vi "手指弯曲.vi"(8 "error in (no error)":errorcluster caption="错误输入（无错误）", 10 "Hands Data In":T1={"手腕"=254.32835, "小手指"=0.0, "无名指"=0.0, "中指"=0.0, "食指"=61.343285, "上下移动"=-1.8918918918918917, "背景色"=15204350, "拇指"=0.0, "转台"=223.8806, "手臂"=20.597015} {"手臂" scale=0.0..90.0; "转台" scale=0.0..360.0; "拇指" scale=0.0..90.0; "上下移动" scale=0.0..100.0; "食指" scale=0.0..90.0; "中指" scale=0.0..90.0; "无名指" scale=0.0..90.0; "小手指" scale=0.0..90.0; "手腕" scale=0.0..360.0}, 11 "Hands Ref In":T2) -> (0 "error out":errorcluster caption="错误输出", 2 "Hands Data Out":T1={"手腕"=52.38806, "小手指"=0.0, "无名指"=0.0, "中指"=0.0, "食指"=0.0, "上下移动"=-1.8918918918918917, "背景色"=15204350, "拇指"=0.0, "转台"=52.38806, "手臂"=52.38806} {"手臂" scale=0.0..90.0; "转台" scale=0.0..360.0; "拇指" scale=0.0..90.0; "上下移动" scale=0.0..100.0; "食指" scale=0.0..90.0; "中指" scale=0.0..90.0; "无名指" scale=0.0..90.0; "小手指" scale=0.0..90.0; "手腕" scale=0.0..360.0}, 3 "Hands Ref Out":T2)   [LabVIEW 2016]
uses:
  Controls/handdata.ctl
  Controls/robotdata.ctl
  <vilib>/picture/3D Picture Control/NI_3D Picture Control.lvlib
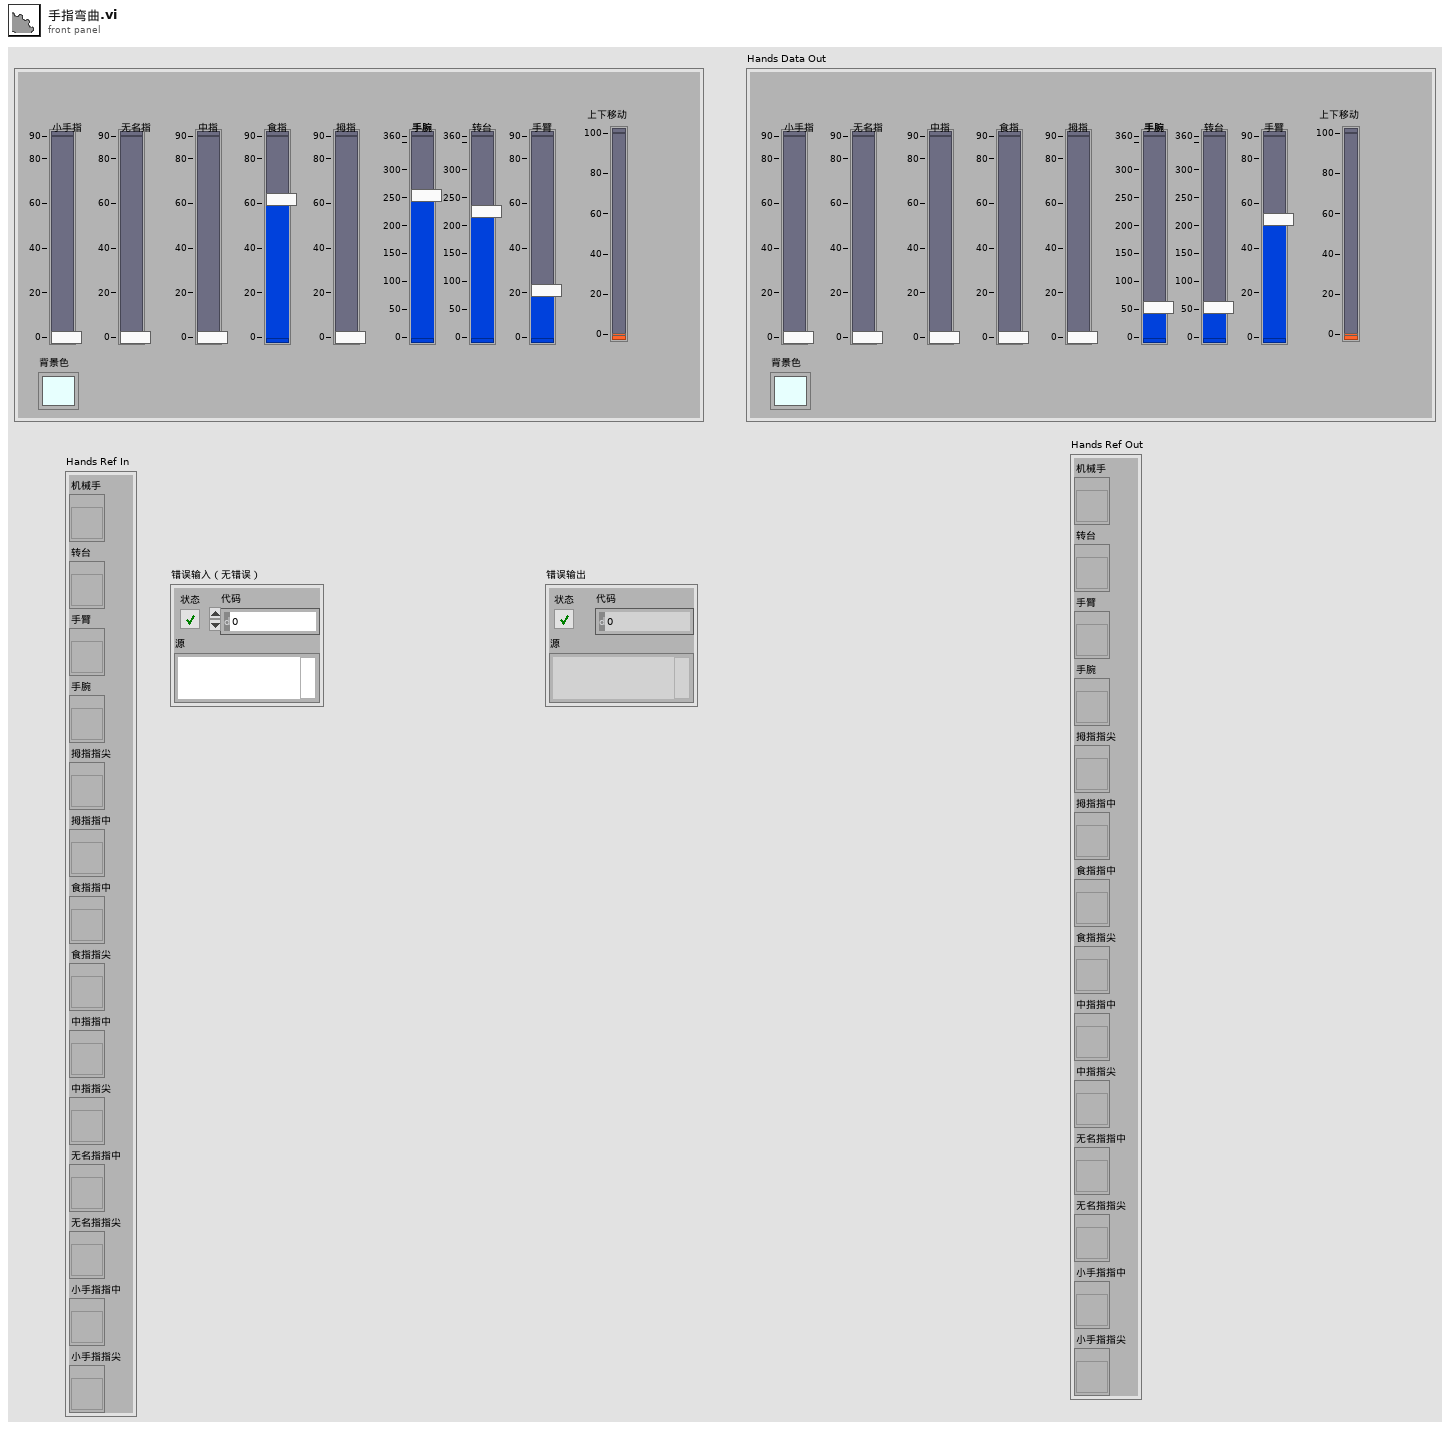
[diagram p1: front panel]
types:
  T1 = typedef "robotdata.ctl" = cluster{"手腕":sgl, "小手指":sgl, "无名指":sgl, "中指":sgl, "食指":sgl, "上下移动":dbl, "背景色":u32, "拇指":sgl, "转台":sgl, "手臂":sgl}
  T2 = typedef "handdata.ctl" = cluster{"机械手":refnum<vi>, "转台":refnum<vi>, "手臂":refnum<vi>, "手腕":refnum<vi>, "拇指指尖":refnum<vi>, "拇指指中 ":refnum<vi>, "食指指中":refnum<vi>, "食指指尖":refnum<vi>, "中指指中":refnum<vi>, "中指指尖":refnum<vi>, "无名指指中":refnum<vi>, "无名指指尖":refnum<vi>, "小手指指中":refnum<vi>, "小手指指尖":refnum<vi>}
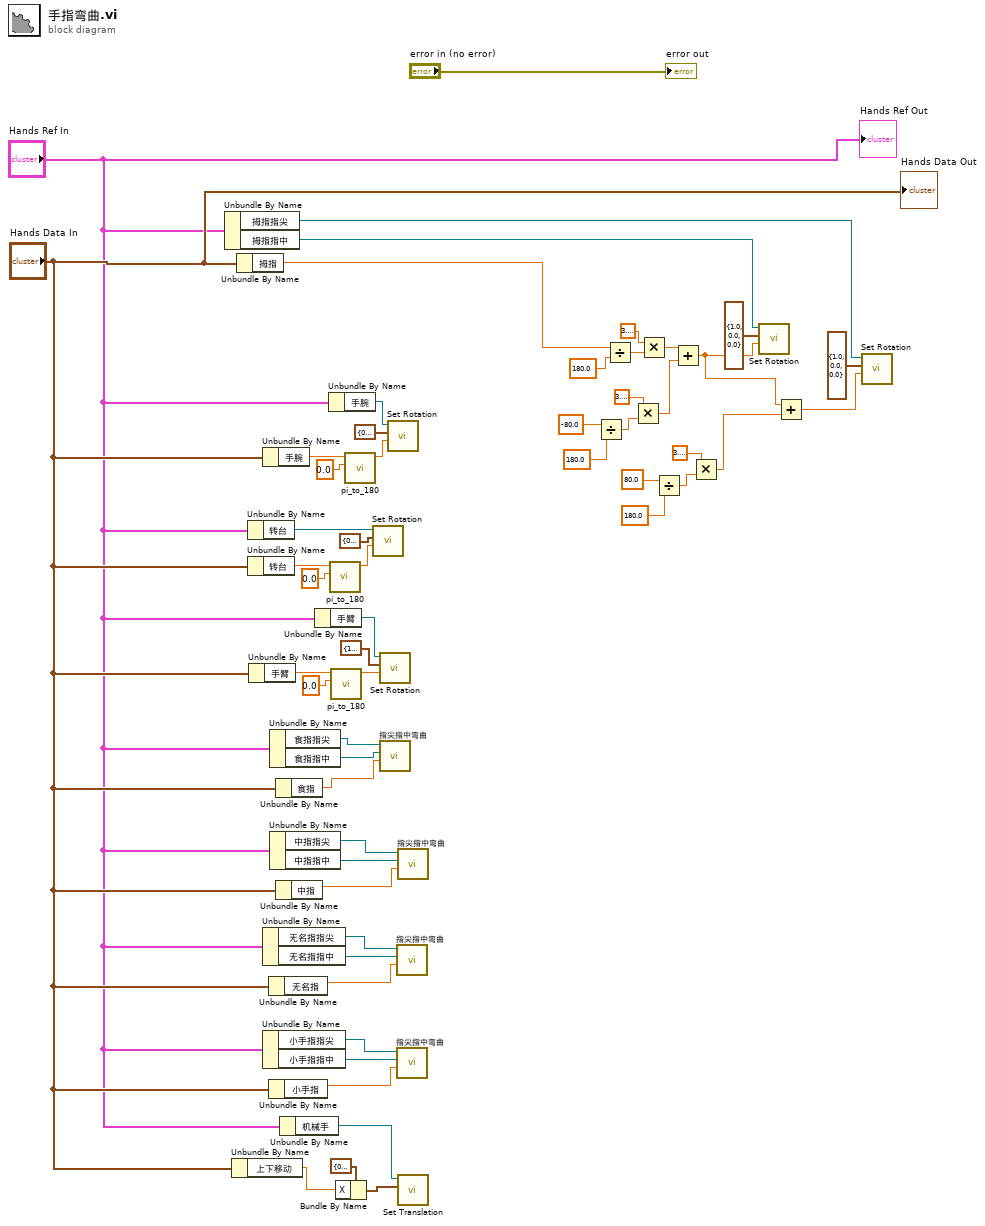
[diagram p0: block diagram]
diagram:
  n1 = Unbundle By Name("Hands Ref In") -> ("拇指指尖"=w10:refnum<vi>, "拇指指中"=w11:refnum<vi>)
  n2 = Unbundle By Name("Hands Data In") -> ("上下移动"=w26:dbl)
  n3 = Unbundle By Name("Hands Data In") -> ("拇指"=w9:sgl)
  n4 = Unbundle By Name("Hands Ref In") -> ("转台"=w49:refnum<vi>)
  n5 = Unbundle By Name("Hands Data In") -> ("转台"=w45:sgl)
  n6 = Unbundle By Name("Hands Data In") -> ("手臂"=w43:sgl)
  n7 = Unbundle By Name("Hands Data In") -> ("手腕"=w51:sgl)
  n8 = Unbundle By Name("Hands Ref In") -> ("无名指指尖"=w34:refnum<vi>, "无名指指中"=w33:refnum<vi>)
  n9 = Unbundle By Name("Hands Ref In") -> ("小手指指尖"=w29:refnum<vi>, "小手指指中"=w30:refnum<vi>)
  n10 = Unbundle By Name("Hands Data In") -> ("无名指"=w32:sgl)
  n11 = Unbundle By Name("Hands Data In") -> ("小手指"=w31:sgl)
  n12 = Unbundle By Name("Hands Ref In") -> ("食指指尖"=w40:refnum<vi>, "食指指中"=w39:refnum<vi>)
  n13 = Unbundle By Name("Hands Ref In") -> ("中指指尖"=w35:refnum<vi>, "中指指中"=w36:refnum<vi>)
  n14 = Unbundle By Name("Hands Data In") -> ("食指"=w38:sgl)
  n15 = Unbundle By Name("Hands Data In") -> ("中指"=w37:sgl)
  n16 = Unbundle By Name("Hands Ref In") -> ("机械手"=w25:refnum<vi>)
  n17 = Unbundle By Name("Hands Ref In") -> ("手臂"=w47:refnum<vi>)
  n18 = Unbundle By Name("Hands Ref In") -> ("手腕"=w52:refnum<vi>)
  n19 = call "pi_to_180.vi"("起始角度"=0.0, "输入角度"=w45) -> ("数值"=w46:dbl)  [unwired: 9 in]
  n20 = call "pi_to_180.vi"("起始角度"=0.0, "输入角度"=w43) -> ("数值"=w41:dbl)  [unwired: 9 in]
  n21 = Bundle By Name(cluster=cluster{"X":sgl, "Y":sgl, "Z":sgl} {"X"=0.0, "Y"=0.0, "Z"=0.0} ("Translation"), "X"=w26) -> (w28:cluster{"X":sgl, "Y":sgl, "Z":sgl})
  n22 = call "pi_to_180.vi"("起始角度"=0.0, "输入角度"=w51) -> ("数值"=w53:dbl)  [unwired: 9 in]
  n23 = call <vilib>:"Set Rotation.vi"("Angle"=w46, "Axis"=cluster{"X":sgl, "Y":sgl, "Z":sgl} {"X"=0.0, "Y"=0.0, "Z"=1.0}, "Scene Object"=w49) -> ()  [unwired: 7 in, 2 out]
  n24 = call <vilib>:"Set Rotation.vi"("Angle"=w41, "Axis"=cluster{"X":sgl, "Y":sgl, "Z":sgl} {"X"=1.0, "Y"=0.0, "Z"=0.0}, "Scene Object"=w47) -> ()  [unwired: 7 in, 2 out]
  n25 = call "指尖指中弯曲.vi"("上限"=w38, "指中"=w39, "指尖"=w40) -> ()  [unwired: 9 in]
  n26 = call <vilib>:"Set Rotation.vi"("Angle"=w53, "Axis"=cluster{"X":sgl, "Y":sgl, "Z":sgl} {"X"=0.0, "Y"=0.0, "Z"=1.0}, "Scene Object"=w52) -> ()  [unwired: 7 in, 2 out]
  n27 = call "指尖指中弯曲.vi"("上限"=w32, "指中"=w33, "指尖"=w34) -> ()  [unwired: 9 in]
  n28 = call "指尖指中弯曲.vi"("上限"=w31, "指中"=w30, "指尖"=w29) -> ()  [unwired: 9 in]
  n29 = call "指尖指中弯曲.vi"("上限"=w37, "指中"=w36, "指尖"=w35) -> ()  [unwired: 9 in]
  n30 = call <vilib>:"Set Translation.vi"("Translation"=w28, "Scene Object"=w25) -> ()  [unwired: 8 in, 2 out]
  n31 = Divide(x=-80.0 ("起始角度 2"), y=180.0) -> (x/y=w18:dbl)
  n32 = Divide(x=w9, y=180.0) -> (x/y=w14:dbl)
  n33 = Multiply(x=3.141592653589793, y=w18) -> (x*y=w20:dbl)
  n34 = Multiply(x=3.141592653589793, y=w14) -> (x*y=w16:dbl)
  n35 = Divide(x=80.0 ("起始角度"), y=180.0) -> (x/y=w6:dbl)
  n36 = Add(x=w16, y=w20) -> (x+y=w4:dbl)
  n37 = Multiply(x=3.141592653589793, y=w6) -> (x*y=w2:dbl)
  n38 = call <vilib>:"Set Rotation.vi"("Angle"=w4, "Axis"=cluster{"X":sgl, "Y":sgl, "Z":sgl} {"X"=1.0, "Y"=0.0, "Z"=0.0}, "Scene Object"=w11) -> ()  [unwired: 7 in, 2 out]
  n39 = Add(x=w4, y=w2) -> (x+y=w3:dbl)
  n40 = call <vilib>:"Set Rotation.vi"("Angle"=w3, "Axis"=cluster{"X":sgl, "Y":sgl, "Z":sgl} {"X"=1.0, "Y"=0.0, "Z"=0.0}, "Scene Object"=w10) -> ()  [unwired: 7 in, 2 out]
  "Hands Ref Out" <- "Hands Ref In"
  "Hands Data Out" <- "Hands Data In"
  "error out" <- "error in (no error)"
